vi "Execution timer.vi"(9 "error in (no error)":errorcluster, 10 "millisecond timer value":u32) -> (1 "error out":errorcluster, 2 "Current or Duration [ms]":u32)   [LabVIEW 2020, in "Broadcast Event Dequeuers.lvlib"]
doc: "Returns the current time in milliseconds if the input is not wired.\nIf the input is wired the time differens is returned in milliseconds."
uses:
  Broadcast Event Dequeuers.lvlib
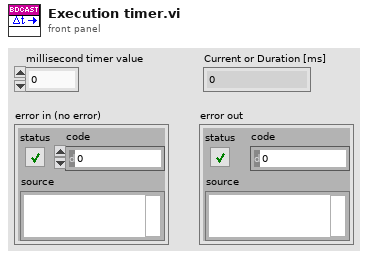
[diagram p1: front panel]
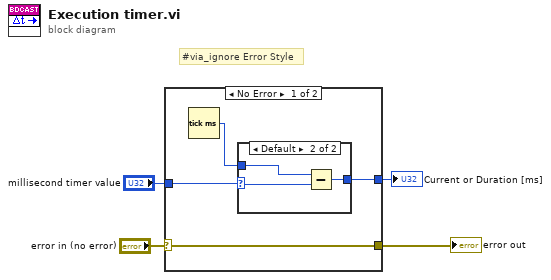
[diagram p0: block diagram]
diagram:
  # "#via_ignore Error Style"
  n1 = case shown="No Error" "error in (no error)" {
    selector: "error in (no error)" -> [w8 w13]
    tunnel: [w8 w13] -> w3
    tunnel: [w5 w14] -> w1
    tunnel: "millisecond timer value" -> [w7 w14]
    frame No Error {
      n2 = Tick Count (ms)() -> (millisecond timer value=w6:u32)
      n3 = case shown="Default" w7 {
        selector: w7 -> [_ w12]
        tunnel: w6 -> [w9 w11]
        tunnel: [w9 w10] -> w5
        frame 0 {
        }
        frame Default {
          n4 = Subtract(x=w11, y=w12) -> (x-y=w10:u32)
        }
      }
    }
    frame Error {
    }
  }
  "error out" <- w3
  "Current or Duration [ms]" <- w1
